vi "EXPRESS Launcher.vi"() -> ()   [LabVIEW 2010]
uses:
  Ctrls/Precess Meter.ctl
  Ctrls/PlotGraph.ctl
  Ctrls/ChannelData.ctl
  Ctrls/ChannelType.ctl
  Ctrls/ChannelAccessType.ctl
  Ctrls/ServerData.ctl
  Ctrls/DeviceInfomation.ctl
  Ctrls/DeviceModel.ctl
  Drivers/ModbusServer/MonitorServer.lvlib
panel:
  in  "剖面管理":bool
  in  "参数配置":bool
  in  "试验箱选择":i32(listbox)
  out "Waveform Graph":T1
  in  "ProcessMeter 4":T2 {"设定值" format="%07.2f"; "当前值" format="%07.2f"}
  in  "ProcessMeter 3":T2 {"设定值" format="%07.2f"; "当前值" format="%07.2f"}
  in  "ProcessMeter 2":T2 {"设定值" format="%07.2f"; "当前值" format="%07.2f"}
  in  "ProcessMeter 1":T2 {"设定值" format="%07.2f"; "当前值" format="%07.2f"}
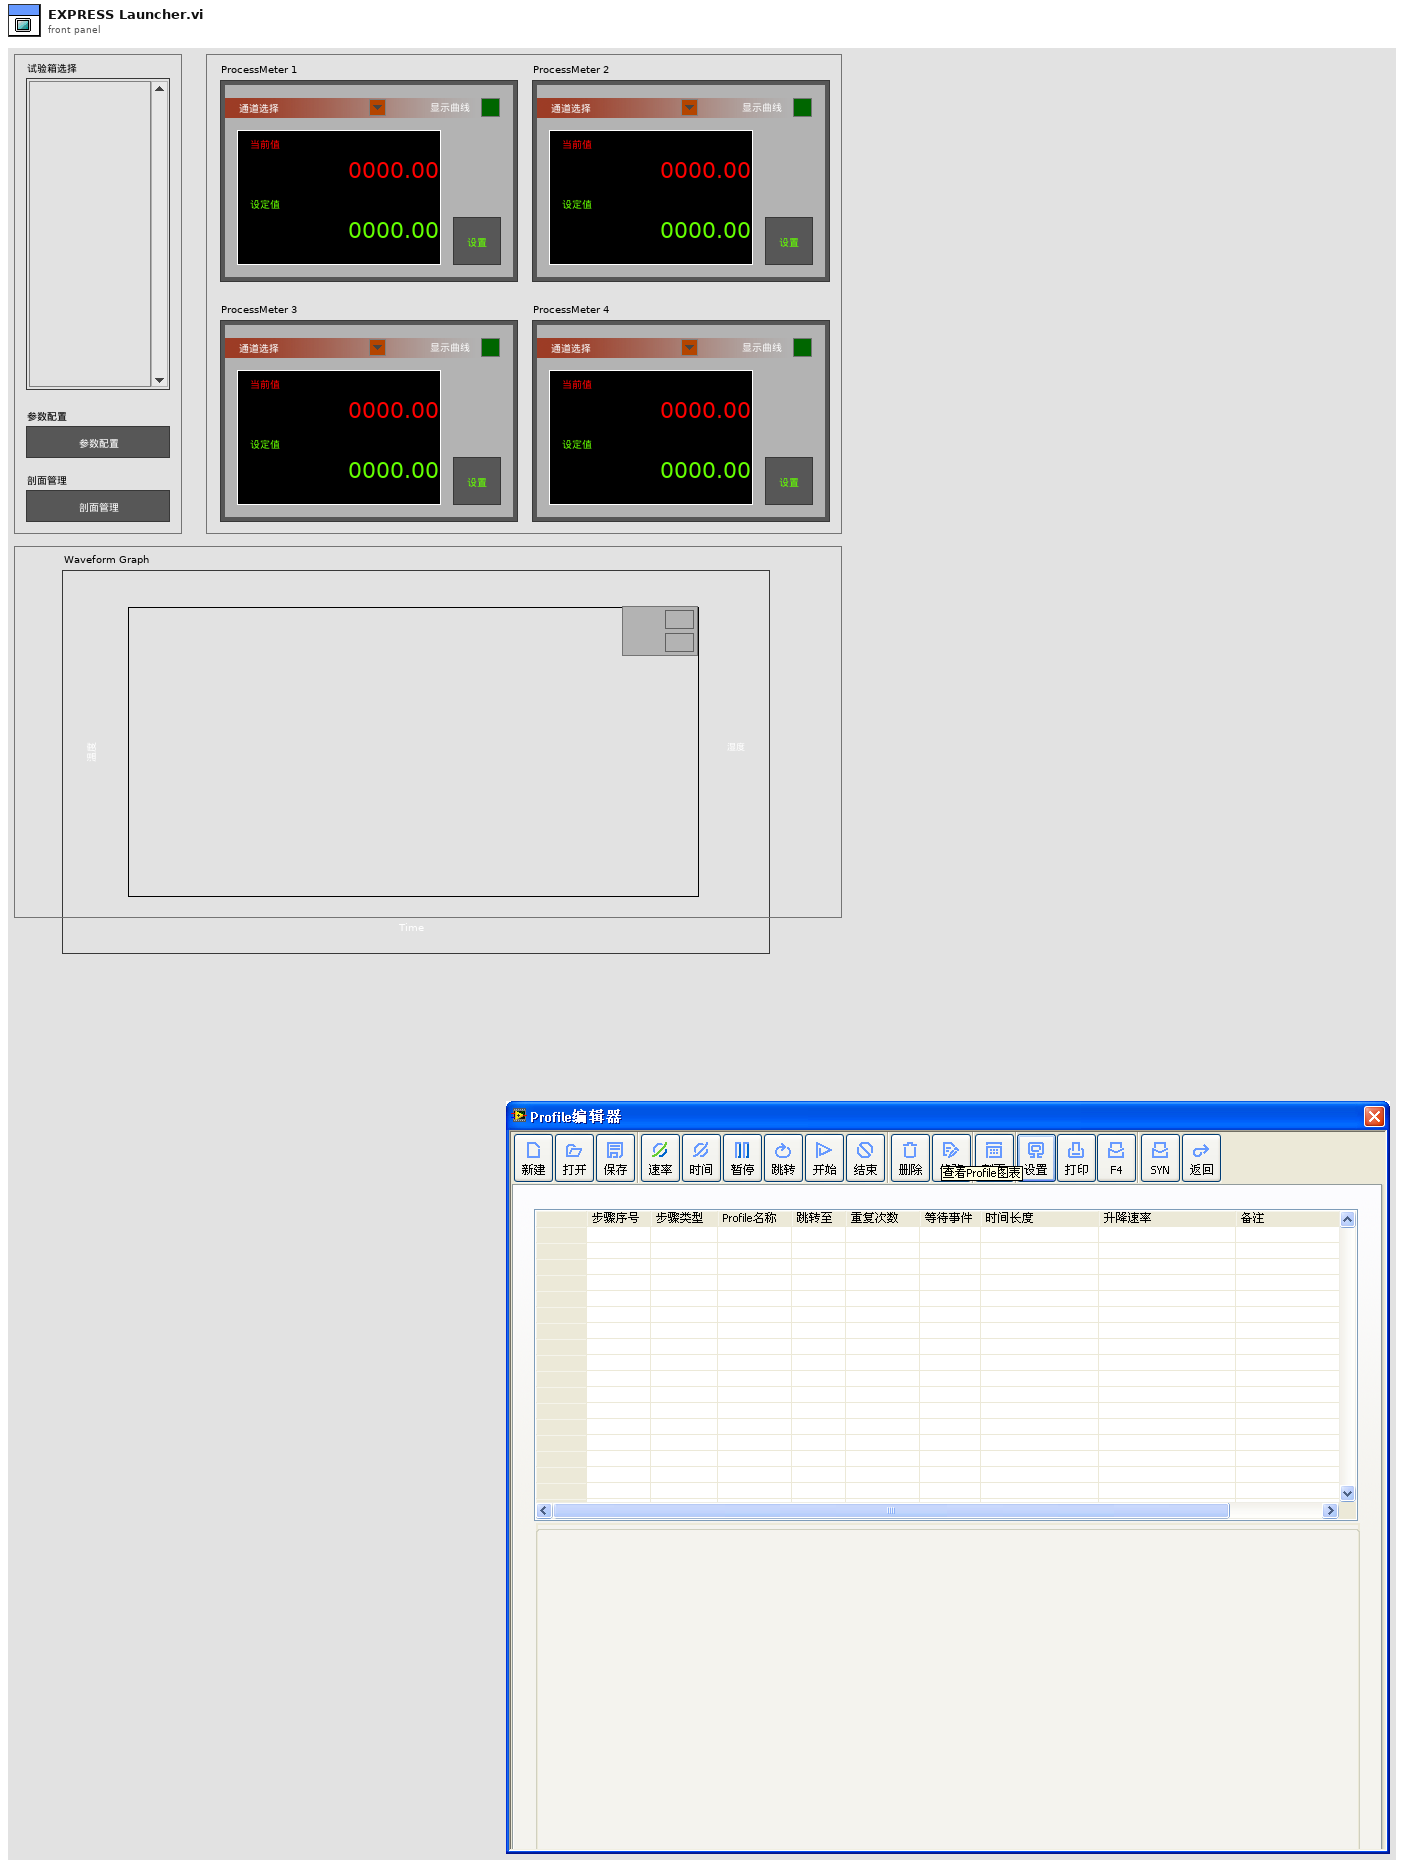
[diagram p1: front panel]
types:
  T1 = typedef "PlotGraph.ctl" = dbl[]
  T2 = typedef "Precess Meter.ctl" = cluster{"当前值":dbl, "设定值":dbl, "通道选择":string, "设置设定值":bool, "显示曲线":bool}
  T3 = enum8{"Enabled", "Disabled", "Disabled and Grayed Out"}
  T4 = enum32{"invalid app kind", "Development System", "Run Time System", "Student Edition", "Embedded LabVIEW", "Evaluation", "Custom"}
  T5 = typedef "ServerData.ctl" = T6[]
  T6 = typedef "DeviceInfomation.ctl" = cluster{"Model":T7, "ChamberName":string, "ChannelNumber":i32, "ChannelsData":T8[], "Connected":bool}
  T7 = typedef "DeviceModel.ctl" = enum16{"WatlowF4", "CenterOne", "DCP551", "DPR250"}
  T8 = typedef "ChannelData.ctl" = cluster{"ChannelName":string, "ChannelType":T9, "AccessType":T10, "ProcessValue":dbl, "SetValue":dbl, "NewSettValue":dbl, "SetNewTarget":bool}
  T9 = typedef "ChannelType.ctl" = enum16{"Temperature", "Humidity"}
  T10 = typedef "ChannelAccessType.ctl" = enum16{"ReadOnly", "SetTarget"}
  T11 = enum32{"Invalid", "Standard", "Closed", "Hidden", "Minimized", "Maximized"}
  T12 = cluster{"Core":cluster{"Current VI Reference":refnum<vi>, "Close Panel on Exit?":bool}, "SelectedDeviceChannelsData":T8[], "试验箱选择ref":refnum<vi>, "通道选择ref":refnum<vi>[], "ProcessMeterRef":refnum<vi>[]}
  T13 = cluster{"Current VI Reference":refnum<vi>, "Close Panel on Exit?":bool}
  T14 = typedef "Path InitDynamicVIsPaths__FS.ctl" = cluster{"F4 Operation":path, "F4 Alarms":path, "F4 Inputs":path, "F4 Outputs":path, "F4 PID Sets":path, "F4 Cascade":path, "F4 Current Step":path, "Profile SubPanel":path, "Profile Editor":path, "MainVI":path, "Profile Control":path, "Synergy Control":path, "Driver Server":path}
  T15 = typedef "Path InitPaths__FS.ctl" = cluster{"Ctrller CFG":path, "INI":path, "Profile":path, "EventLog":path, "Data":path}
  T16 = typedef "Controller Configuration__CHC.ctl" = cluster{"Ctrller Type":T17, "Ctrller Name":string, "Ctrller Addr":string, "Server IP":string, "Conn Result":string, "Port":string, "Baud":dbl}
  T17 = typedef "Controller Configuration__Ctrller Type.ctl" = enum16{"F4S/D", "Synergy"}
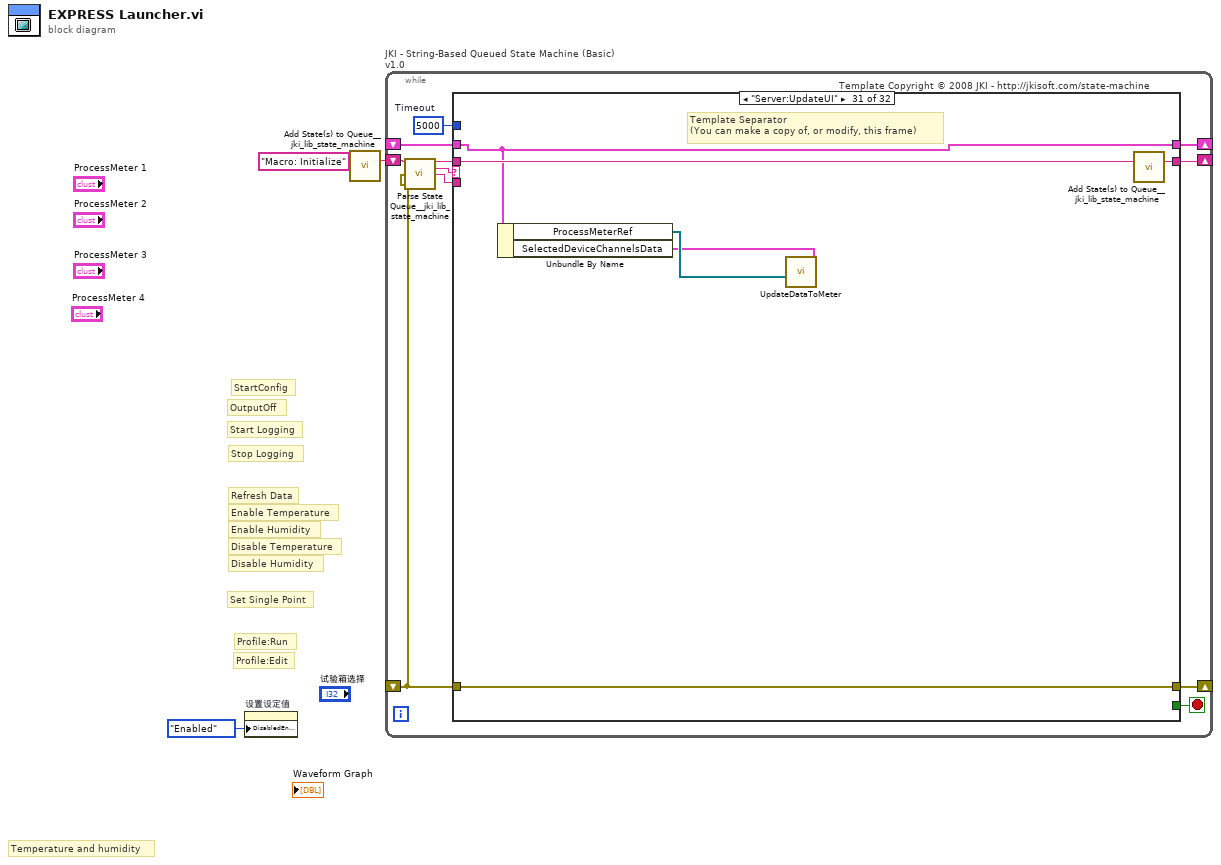
[diagram p0: block diagram]
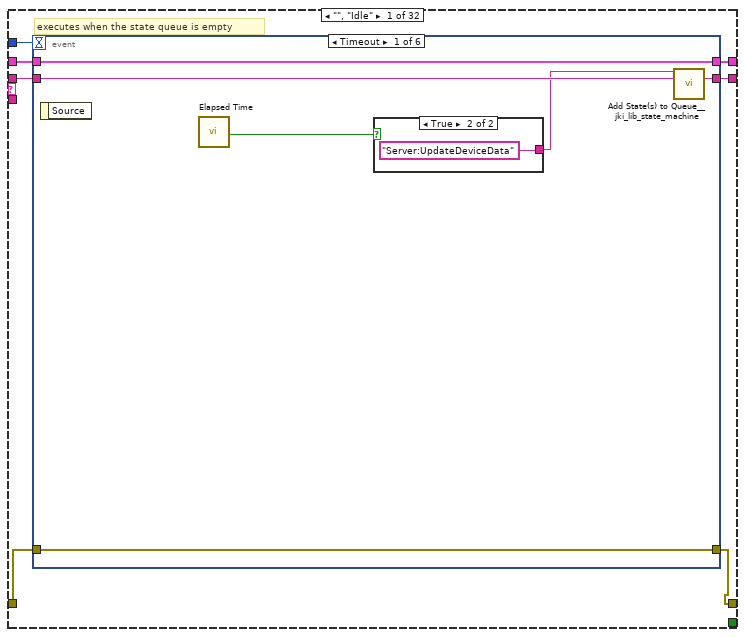
[diagram p2: hidden frame]
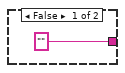
[diagram p3: hidden frame]
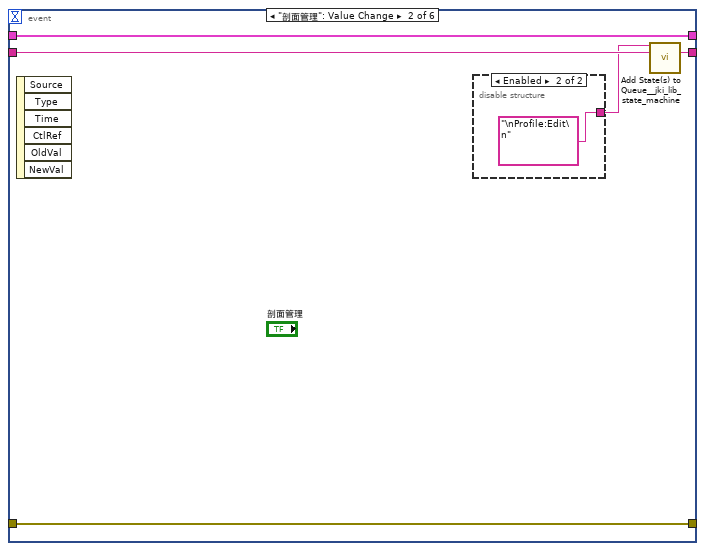
[diagram p4: hidden frame]
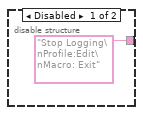
[diagram p5: hidden frame]
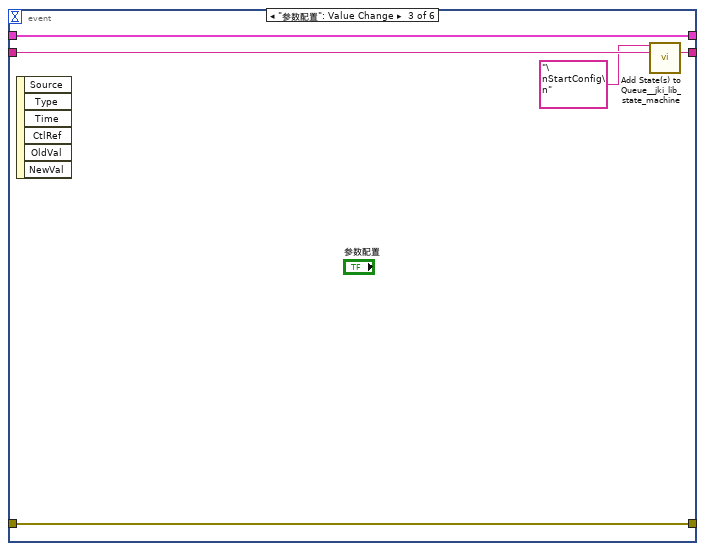
[diagram p6: hidden frame]
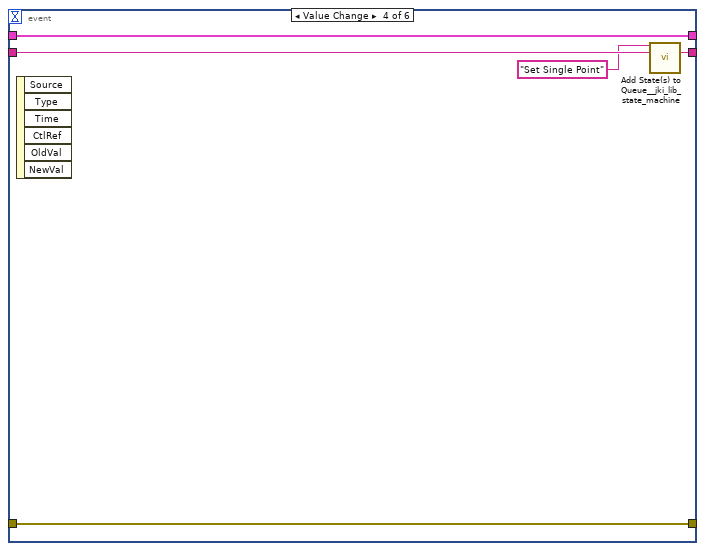
[diagram p7: hidden frame]
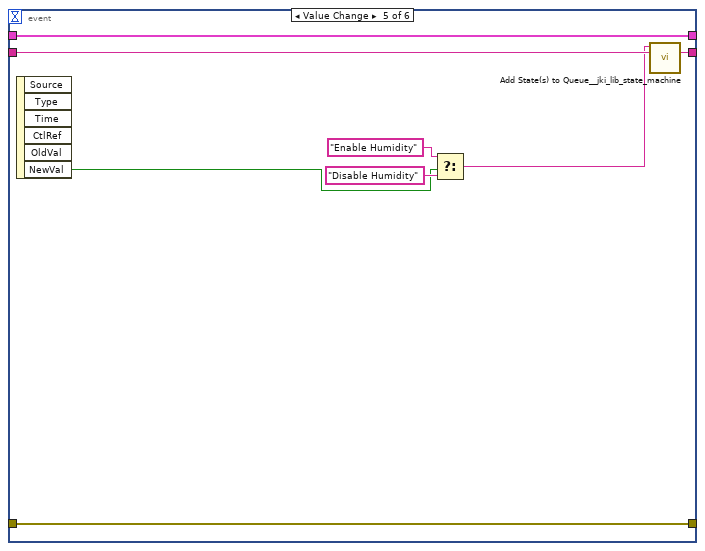
[diagram p8: hidden frame]
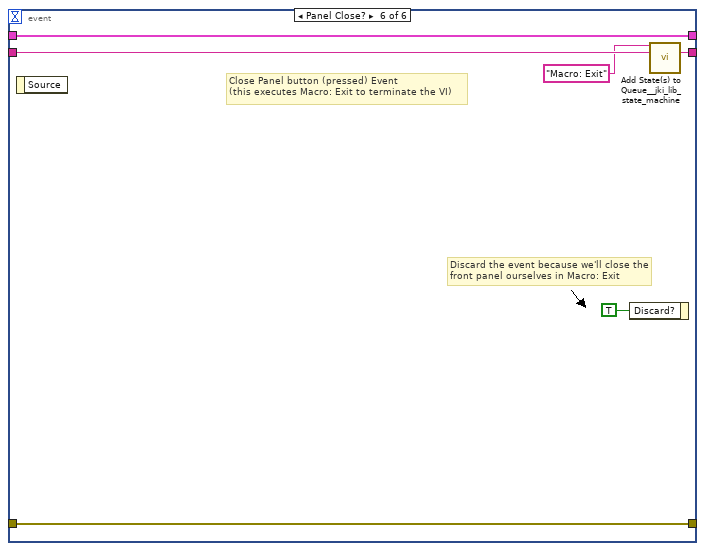
[diagram p9: hidden frame]
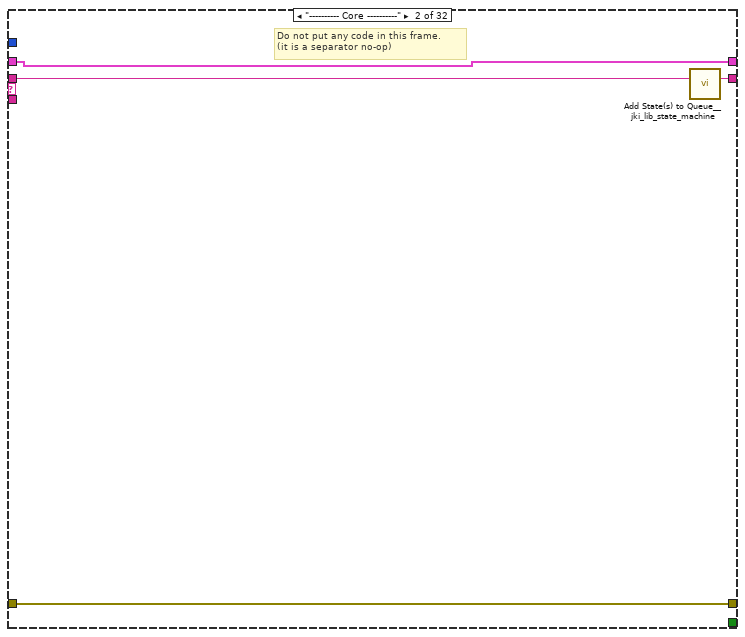
[diagram p10: hidden frame]
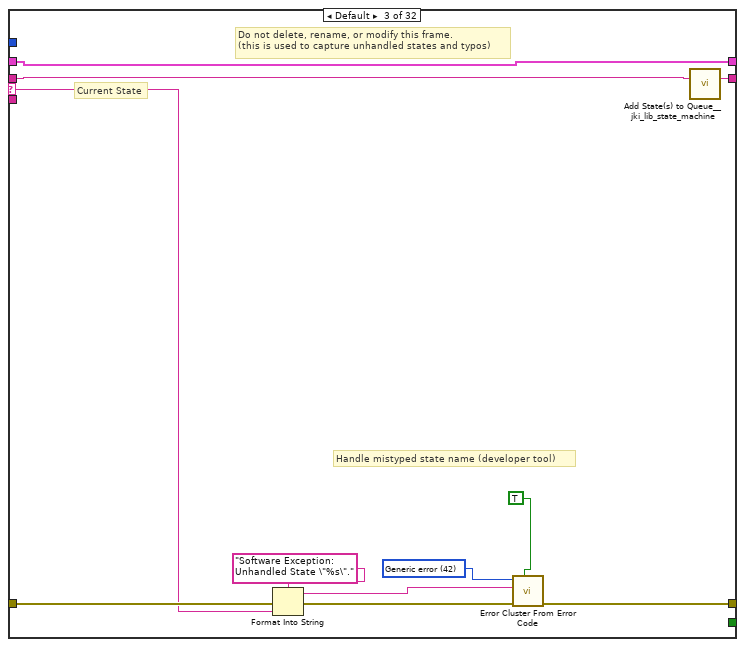
[diagram p11: hidden frame]
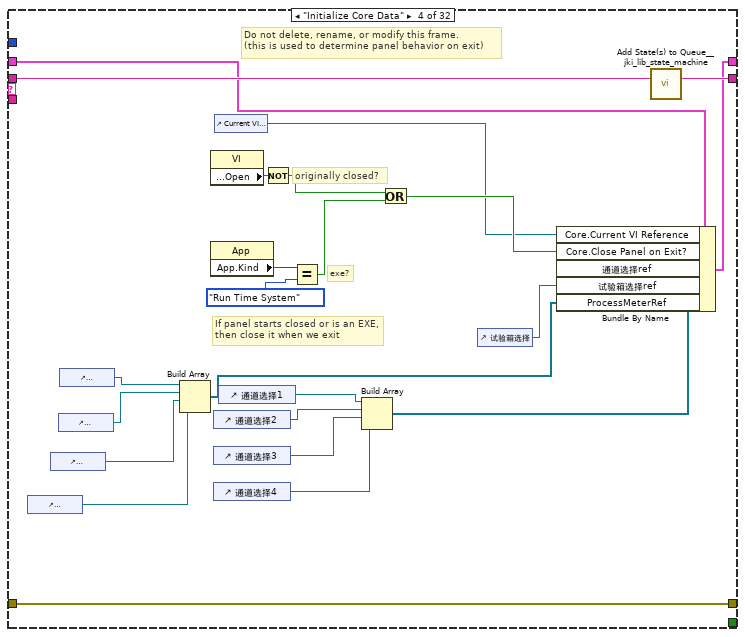
[diagram p12: hidden frame]
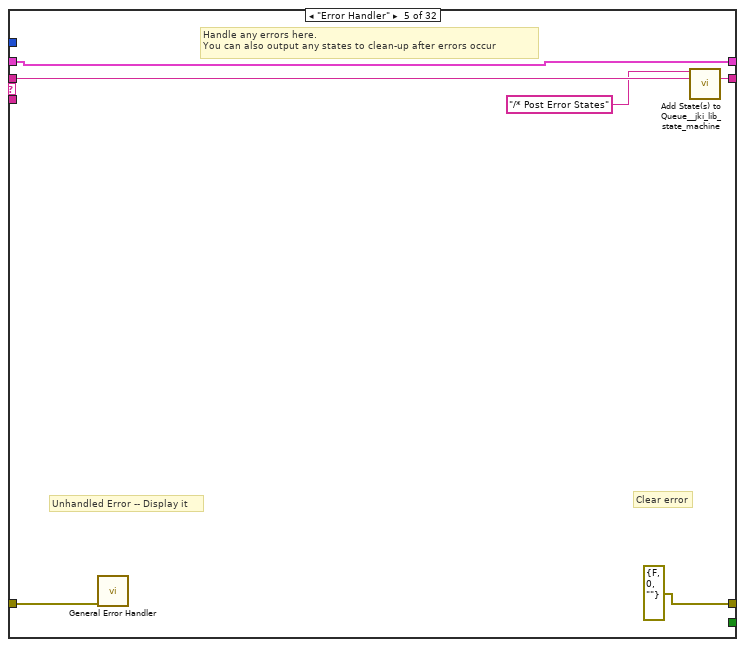
[diagram p13: hidden frame]
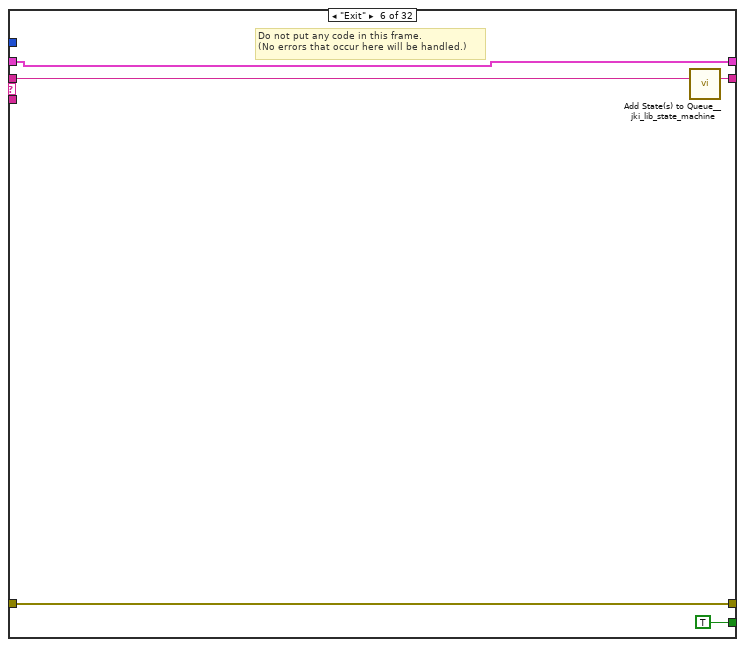
[diagram p14: hidden frame]
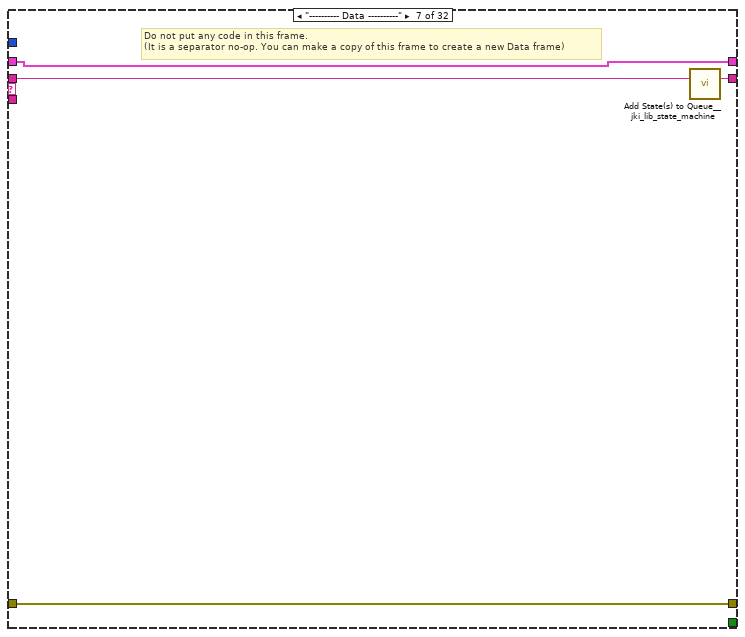
[diagram p15: hidden frame]
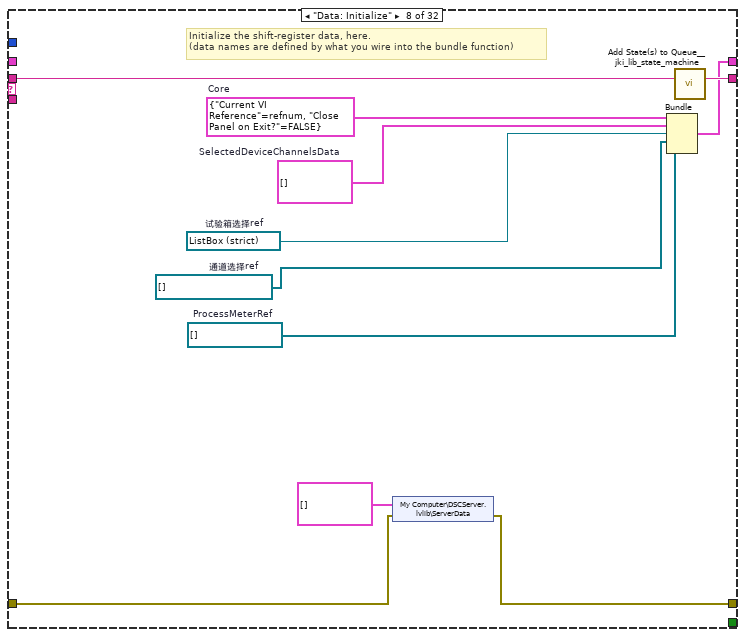
[diagram p16: hidden frame]
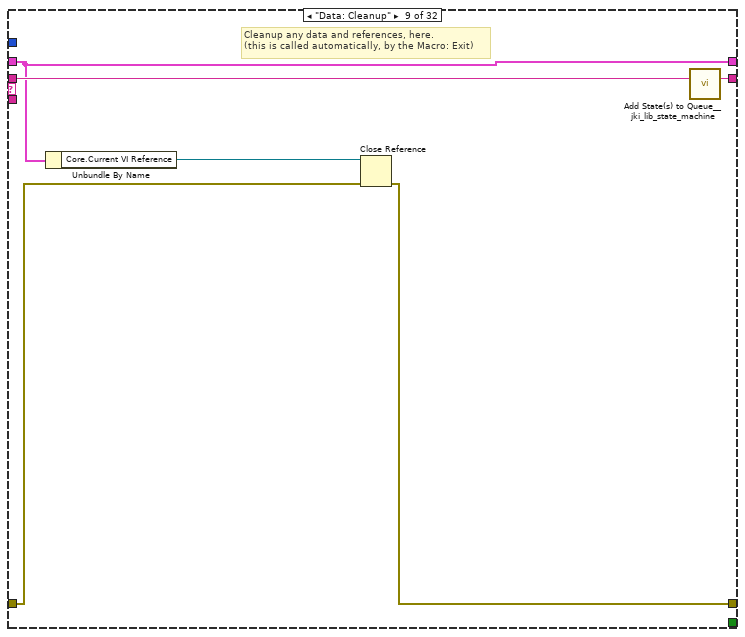
[diagram p17: hidden frame]
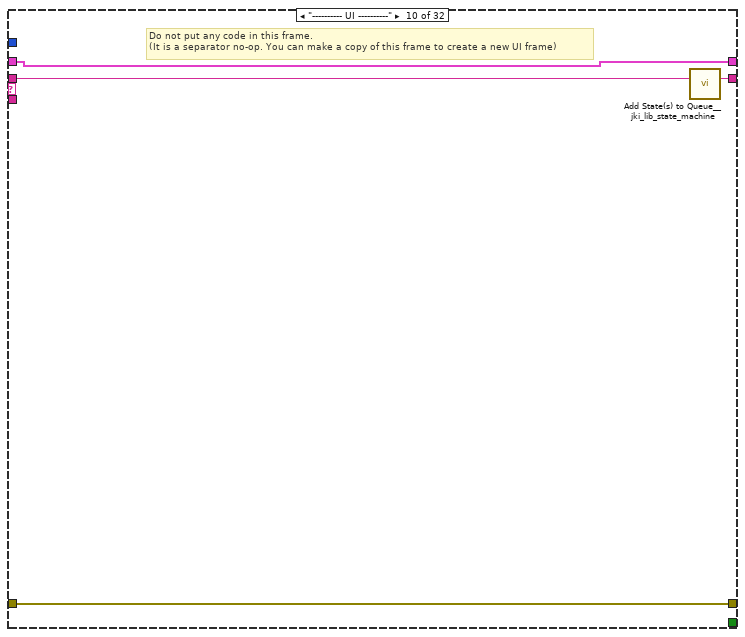
[diagram p18: hidden frame]
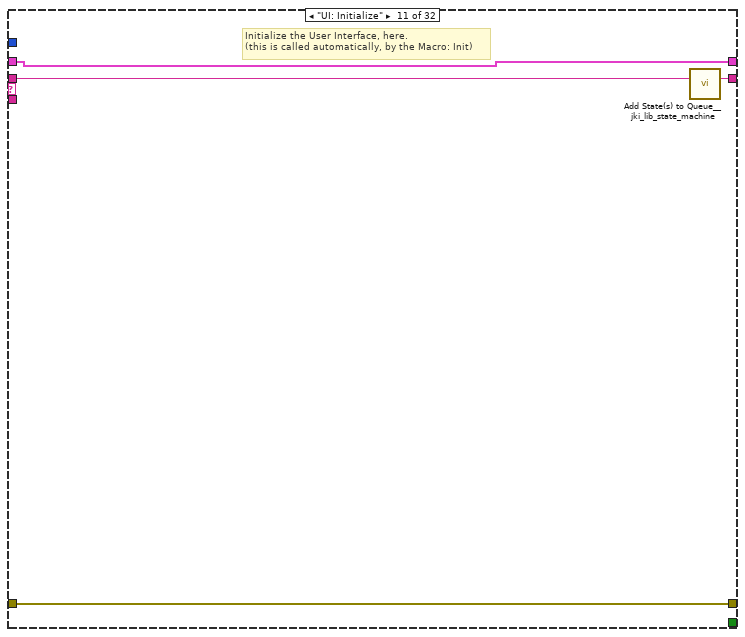
[diagram p19: hidden frame]
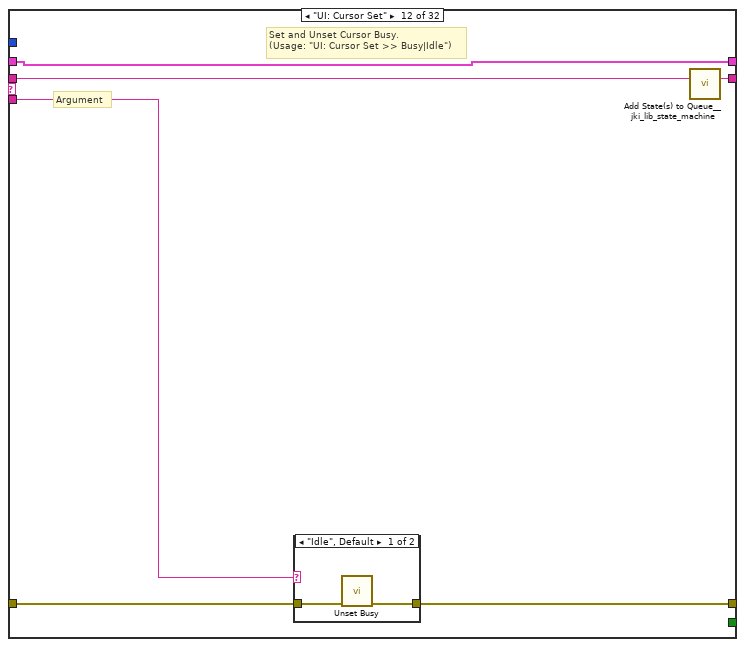
[diagram p20: hidden frame]
diagram:
  # "StartConfig"
  # "OutputOff"
  # "Profile:Edit"
  # "Profile:Run"
  # "Set Single Point"
  # "Stop Logging"
  # "Start Logging"
  # "Disable Humidity"
  # "Disable Temperature"
  # "Enable Temperature"
  # "Refresh Data"
  # "Enable Humidity"
  # "Temperature and humidity"
  n1 = property on="设置设定值" class="Bool"("DisabledEnum"=T3."Enabled" ("Disabled")) -> ()  [unwired: 2 in, 2 out]
  n2 = call "Add State(s) to Queue__jki_lib_state_machine.vi"("State(s) in (\"\")"="Macro: Initialize") -> ("States Out"=w3:string)  [unwired: 14 in]
  n3 = while "JKI - String-Based Queued State Machine (Basic) v1.0" {
    shift-right: [w7] -> _
    shift-left: _ -> [w6]
    shift-right: [w10] -> _
    shift-left: _ -> [w4]
    shift-right: [w9] -> _
    shift-left: w3 -> [w11]
    stop <- w8 stop-if-true
    w5 = 5000  # Timeout
    # "Template Copyright © 2008 JKI - http://jkisoft.com/state-machine"
    n4 = call "Parse State Queue__jki_lib_state_machine.vi"("State Queue"=w11, "Error In (no error)"=w4) -> ("Remaining States"=w13:string, "Current State"=w14:string, "Arguments"=w12:string)  [unwired: 11 in]
    n5 = case shown="\"Server:UpdateUI\"" w14 {
      selector: w14 -> [_ _ w65 _ _ _ _ _ _ _ _ _ _ _ _ _ _ _ _ _ _ _ _ _ _ _ _ _ _ _ _ _]
      tunnel: w13 -> [w21 w64 w69 w98 w104 w109 w113 w124 w130 w134 w138 w144 w155 w181 w186 w196 w200 w209 w214 w219 w227 w231 w236 w252 w257 w261 w265 w269 w273 w277 w283 w294]
      tunnel: w12 -> [_ _ _ _ _ _ _ _ _ _ _ w139 w149 _ _ _ _ _ _ _ _ _ _ _ _ _ _ _ _ _ _ _]
      tunnel: w6 -> [w19 w61 w67 w89 w101 w107 w110 _ w125 w131 w136 w142 w151 w178 w183 w193 w197 w207 w212 w217 w224 w228 w234 w250 w255 w259 w263 w267 w271 w274 w280 w291]
      tunnel: [w18 w62 w71 w95 errorcluster {"status"=FALSE, "code"=0, "source"=""} ("error out") w106 w111 w118 w126 w132 w135 w140 w152 w179 w184 w194 w198 w201 w210 w215 w225 w229 w232 w237 w253 w258 w262 w266 w270 w275 w281 w284] -> w10
      tunnel: w4 -> [w17 w62 w70 w95 w100 w106 w111 w119 w127 w132 w135 w141 w153 w179 w184 w194 w198 w202 w211 w216 w225 w229 w233 w241 w254 w258 w262 w266 w270 w275 w281 w285]
      tunnel: [w20 w63 w68 w97 w103 w108 w112 w123 w129 w133 w137 w143 w154 w180 w185 w195 w199 w208 w213 w218 w226 w230 w235 w251 w256 w260 w264 w268 w272 w276 w282 w293] -> w9
      tunnel: [_ _ _ _ _ TRUE _ _ _ _ _ _ _ _ _ _ _ _ _ _ _ _ _ _ _ _ _ _ _ _ _ _] -> w8
      tunnel: [w16 w61 w67 w96 w101 w107 w110 w122 w125 w131 w136 w142 w151 w178 w183 w193 w197 w207 w212 w217 w224 w228 w234 w250 w255 w259 w263 w267 w271 w274 w280 w287] -> w7
      tunnel: w5 -> [w15 _ _ _ _ _ _ _ _ _ _ _ _ _ _ _ _ _ _ _ _ _ _ _ _ _ _ _ _ _ _ _]
      frame "", "Idle" {
        # "executes when the state queue is empty"
        n6 = event shown="[0] Timeout" {
          selector: _ -> [_ _ _ _ _ _]
          dyn-events: _ -> [_ _ _ _ _ _]
          timeout: w15 -> [_ _ _ _ _ _]
          tunnel: w21 -> [w27 w34 w41 w46 w54 w60]
          tunnel: [w26 w33 w40 w45 w53 w59] -> w20
          tunnel: w19 -> [w24 w31 w38 w43 w51 w57]
          tunnel: [w25 w32 w39 w44 w52 w58] -> w18
          tunnel: w17 -> [w25 w32 w39 w44 w52 w58]
          tunnel: [w24 w31 w38 w43 w51 w57] -> w16
          event Timeout {
            n7 = event-data() -> ()  [unwired: 1 in, 1 out]
            n8 = call "Elapsed Time"() -> ("Time has Elapsed"=w23:bool)  [unwired: 12 in, 7 out]
            n9 = case shown="True" w23 {
              tunnel: ["" ("State(s) in Front (\"\")") "Server:UpdateDeviceData" ("State(s) in Front (\"\")")] -> w22
              frame False {
              }
              frame True {
              }
            }
            n10 = call "Add State(s) to Queue__jki_lib_state_machine.vi"("State(s) in Front (\"\")"=w22, "State(s) in (\"\")"=w27) -> ("States Out"=w26:string)  [unwired: 13 in]
          }
          event "剖面管理": Value Change {
            n11 = event-data() -> ()  [unwired: 1 in, 6 out]
            n12 = disable-structure shown="Enabled" {
              disable-tunnel: ["Stop Logging\nProfile:Edit\nMacro: Exit" ("State(s) in Front (\"\")") "\nProfile:Edit\n" ("State(s) in Front (\"\")")] -> w30
              frame Disabled {
              }
              frame Enabled {
              }
            }
            n13 = call "Add State(s) to Queue__jki_lib_state_machine.vi"("State(s) in Front (\"\")"=w30, "State(s) in (\"\")"=w34) -> ("States Out"=w33:string)  [unwired: 13 in]
          }
          event "参数配置": Value Change {
            n14 = event-data() -> ()  [unwired: 1 in, 6 out]
            n15 = call "Add State(s) to Queue__jki_lib_state_machine.vi"("State(s) in Front (\"\")"="\nStartConfig\n" ("State(s) in Front (\"\")"), "State(s) in (\"\")"=w41) -> ("States Out"=w40:string)  [unwired: 13 in]
          }
          event Value Change {
            n16 = event-data() -> ()  [unwired: 1 in, 6 out]
            n17 = call "Add State(s) to Queue__jki_lib_state_machine.vi"("State(s) in Front (\"\")"="Set Single Point" ("State(s) in Front (\"\")"), "State(s) in (\"\")"=w46) -> ("States Out"=w45:string)  [unwired: 13 in]
          }
          event Value Change {
            n18 = event-data() -> ("NewVal"=w47:bool)  [unwired: 1 in, 5 out]
            n19 = Select(t="Enable Humidity" ("State(s) in Front (\"\")"), s=w47, f="Disable Humidity") -> (s? t:f=w48:string)
            n20 = call "Add State(s) to Queue__jki_lib_state_machine.vi"("State(s) in Front (\"\")"=w48, "State(s) in (\"\")"=w54) -> ("States Out"=w53:string)  [unwired: 13 in]
          }
          event Panel Close? {
            # "Discard the event because we'll close the front panel ourselves in Macro: Exit"
            # "Close Panel button (pressed) Event\n(this executes Macro: Exit to terminate the VI)"
            n21 = event-data() -> ()  [unwired: 1 in, 1 out]
            n22 = event-data("Discard?"=TRUE) -> ()  [unwired: 1 in, 1 out]
            n23 = call "Add State(s) to Queue__jki_lib_state_machine.vi"("State(s) in Front (\"\")"="Macro: Exit", "State(s) in (\"\")"=w60) -> ("States Out"=w59:string)  [unwired: 13 in]
          }
        }
      }
      frame "---------- Core ----------" {
        # "Do not put any code in this frame.\n(it is a separator no-op)"
        n24 = call "Add State(s) to Queue__jki_lib_state_machine.vi"("State(s) in (\"\")"=w64) -> ("States Out"=w63:string)  [unwired: 14 in]
      }
      frame Default {
        w74 = 42 items=["No error", "Argument error", "Memory is full", "Out of zone", "End of file", "File already open", "Generic file I/O error", "File not found", "File permission error", "Disk is full", "Duplicate path", "Too many files open", "System feature not enabled", "Resource file not found", "Cannot add resource", "Resource not found", "Image not found", "Image memory error", "Pen does not exist", "Config type invalid", "Config token not found", "Config parse error", "Config memory error", "Bad external code format", "Bad external code offset", "External code not present", "Null window", "Destroy window error", "Null menu", "Print aborted", "Bad print record", "Print driver error", "Windows error during printing", "Memory error during printing", "Print dialog error", "Generic print error", "Invalid device refnum", "Device not found", "Device parameter error", "Device unit error", "Cannot open device", "Device call aborted", "Generic error", "Cancelled by user", "Object ID too low", "Object ID too high", "Object not in heap", "Unknown heap", "Unknown object (invalid DefProc)", "Unknown object (DefProc not in table)", "Message out of range", "Invalid (null) method", "Unknown message", "Manager call not supported", "Bad address", "Network operation in progress", "Network operation timed out", "Connection is busy", "Network attribute not supported", "Network error", "Address in use", "System out of memory", "Connection aborted", "Connection refused", "Not connected", "Already connected", "Connection closed", "Initialization error (interapplication manager)", "Bad occurrence", "Wait on unbound occurrence handler", "Occurrence queue overflow", "Datalog type conflict", "Unused", "Unrecognized type (interapplication manager)", "Memory corrupt", "Failed to make temporary DLL", "Old CIN version", "Drag socket not found", "Failed to load drop-object", "Failed to register OLE object", "Failed to release OLE object", "Format specifier type mismatch", "Unknown format specifier", "Too few format specifiers", "Too many format specifiers", "Scan failed", "Newer CIN version", "Error converting to variant", "Runtime menu error", "Password tampered", "Variant attribute not found", "Incompatible variant data type", "Event data is not available", "Event Store is not present", "Occurrence is not found", "Event Queue is not created", "Event info is not available", "Refnum passed is NULL", "Error retrieving Class GUID", "Error retrieving CoClass GUID", "Error retrieving TypeLib GUID.", "Bad built application magic bytes.", "Specific driver is different from the specific driver associated with the Logical Name.", "There is no session opened to the class driver.", "Max Error", "MAX - Error with config objects", "MAX - Error loading configuration", "MAX - Group not supported"]
        # "Current State"
        # "Do not delete, rename, or modify this frame.\n(this is used to capture unhandled states and typos)"
        # "Handle mistyped state name (developer tool)"
        n25 = Format Into String(format string="Software Exception: Unhandled State \"%s\"." ("message"), error in=w70, w65) -> (resulting string=w73:string, error out=w72:errorcluster)  [unwired: 1 in]
        n26 = call <vilib>:"Error Cluster From Error Code.vi"("show call chain? (False)"=TRUE, "error in (no error)"=w72, "error message (\"\")"=w73, "error code (0)"=w74) -> ("error out"=w71:errorcluster)  [unwired: 5 in]
        n27 = call "Add State(s) to Queue__jki_lib_state_machine.vi"("State(s) in (\"\")"=w69) -> ("States Out"=w68:string)  [unwired: 14 in]
      }
      frame "Initialize Core Data" {
        # "Do not delete, rename, or modify this frame.\n(this is used to determine panel behavior on exit)"
        # "originally closed?"
        # "exe?"
        # "If panel starts closed or is an EXE, then close it when we exit"
        n28 = control-ref of="ProcessMeter 4"() -> (w77:refnum<vi>)
        n29 = control-ref of="ProcessMeter 3"() -> (w78:refnum<vi>)
        n30 = control-ref of="ProcessMeter 2"() -> (w79:refnum<vi>)
        n31 = control-ref of="ProcessMeter 1"() -> (w80:refnum<vi>)
        n32 = Build Array(w80, w79, w78, w77) -> (w76:refnum<vi>[])
        n33 = property class="VI"() -> ("Front Panel.Open"=w94:bool)  [unwired: 2 in, 2 out]
        n34 = property class="App"() -> ("App.Kind"=w93:T4)  [unwired: 2 in, 2 out]
        n35 = control-ref of="通道选择2"() -> (w85:refnum<vi>)
        n36 = control-ref of="通道选择3"() -> (w84:refnum<vi>)
        n37 = control-ref of="通道选择4"() -> (w83:refnum<vi>)
        n38 = control-ref of="Current VI Reference"() -> (w87:refnum<vi>)
        n39 = control-ref of="通道选择1"() -> (w86:refnum<vi>)
        n40 = Not(x=w94) -> (.not. x?=w91:bool)
        n41 = Equal?(x=w93, y=T4."Run Time System" ("Application:Kind")) -> (x = y?=w90:bool)
        n42 = Build Array(w86, w85, w84, w83) -> (w82:refnum<vi>[])
        n43 = Or(x=w91, y=w90) -> (x .or. y?=w88:bool)
        n44 = control-ref of="试验箱选择"() -> (w81:refnum<vi>)
        n45 = Bundle By Name(cluster=w89, "Core.Current VI Reference"=w87, "Core.Close Panel on Exit?"=w88, "通道选择ref"=w82, "试验箱选择ref"=w81, "ProcessMeterRef"=w76) -> (w96:T12)
        n46 = call "Add State(s) to Queue__jki_lib_state_machine.vi"("State(s) in (\"\")"=w98) -> ("States Out"=w97:string)  [unwired: 14 in]
      }
      frame "Error Handler" {
        # "Unhandled Error -- Display it"
        # "Handle any errors here.\nYou can also output any states to clean-up after errors occur"
        # "Clear error"
        n47 = call <vilib>:"General Error Handler.vi"("error in (no error)"=w100) -> ()  [unwired: 10 in, 5 out]
        n48 = call "Add State(s) to Queue__jki_lib_state_machine.vi"("State(s) in Front (\"\")"="/* Post Error States", "State(s) in (\"\")"=w104) -> ("States Out"=w103:string)  [unwired: 13 in]
      }
      frame "Exit" {
        # "Do not put any code in this frame.\n(No errors that occur here will be handled.)"
        n49 = call "Add State(s) to Queue__jki_lib_state_machine.vi"("State(s) in (\"\")"=w109) -> ("States Out"=w108:string)  [unwired: 14 in]
      }
      frame "---------- Data ----------" {
        # "Do not put any code in this frame.\n(It is a separator no-op. You can make a copy of this frame to create a new Data frame)"
        n50 = call "Add State(s) to Queue__jki_lib_state_machine.vi"("State(s) in (\"\")"=w113) -> ("States Out"=w112:string)  [unwired: 14 in]
      }
      frame "Data: Initialize" {
        w114 = refnum<vi>[] []  # ProcessMeterRef
        w115 = refnum<vi> refnum  # 试验箱选择ref
        w116 = refnum<vi>[] []  # 通道选择ref
        w117 = T8[] []  # SelectedDeviceChannelsData
        w121 = T13 {"Current VI Reference"=refnum, "Close Panel on Exit?"=FALSE}  # Core
        # "Initialize the shift-register data, here.\n(data names are defined by what you wire into the bundle function)"
        n51 = shared-variable "My Computer\\DSCServer.lvlib\\ServerData"(T5 [] ("ServerData"), error in=w119) -> (error out=w118:errorcluster)
        n52 = Bundle("Core"=w121, "SelectedDeviceChannelsData"=w117, "试验箱选择ref"=w115, "通道选择ref"=w116, "ProcessMeterRef"=w114) -> (w122:T12)  [unwired: 1 in]
        n53 = call "Add State(s) to Queue__jki_lib_state_machine.vi"("State(s) in (\"\")"=w124) -> ("States Out"=w123:string)  [unwired: 14 in]
      }
      frame "Data: Cleanup" {
        # "Cleanup any data and references, here.\n(this is called automatically, by the Macro: Exit)"
        n54 = Unbundle By Name(w125) -> ("Core.Current VI Reference"=w128:refnum<vi>)
        n55 = Close Reference(reference=w128, error in (no error)=w127) -> (error out=w126:errorcluster)
        n56 = call "Add State(s) to Queue__jki_lib_state_machine.vi"("State(s) in (\"\")"=w130) -> ("States Out"=w129:string)  [unwired: 14 in]
      }
      frame "---------- UI ----------" {
        # "Do not put any code in this frame.\n(It is a separator no-op. You can make a copy of this frame to create a new UI frame)"
        n57 = call "Add State(s) to Queue__jki_lib_state_machine.vi"("State(s) in (\"\")"=w134) -> ("States Out"=w133:string)  [unwired: 14 in]
      }
      frame "UI: Initialize" {
        # "Initialize the User Interface, here.\n(this is called automatically, by the Macro: Init)"
        n58 = call "Add State(s) to Queue__jki_lib_state_machine.vi"("State(s) in (\"\")"=w138) -> ("States Out"=w137:string)  [unwired: 14 in]
      }
      frame "UI: Cursor Set" {
        # "Argument"
        # "Set and Unset Cursor Busy.\n(Usage: \"UI: Cursor Set >> Busy|Idle\")"
        n59 = case shown="\"Idle\", Default" w139 {
          tunnel: w141 -> [w146 w148]
          tunnel: [w145 w147] -> w140
          frame "Idle", Default {
            n60 = call <vilib>:"Unset Busy.vi"("error in (no error)"=w146) -> ("error out"=w145:errorcluster)  [unwired: 10 in]
          }
          frame "Busy" {
            n61 = call <vilib>:"Set Busy.vi"("error in (no error)"=w148) -> ("error out"=w147:errorcluster)  [unwired: 9 in, 1 out]
          }
        }
        n62 = call "Add State(s) to Queue__jki_lib_state_machine.vi"("State(s) in (\"\")"=w144) -> ("States Out"=w143:string)  [unwired: 14 in]
      }
      frame "UI: Front Panel State" {
        # "Argument"
        # "Set Front Panel Open or Closed\n(Usage: \"UI: Front Panel State >> Open|Close\")"
        n63 = Unbundle By Name(w151) -> ("Core.Current VI Reference"=w150:refnum<vi>)
        n64 = case shown="\"Open\", Default" w149 {
          tunnel: w153 -> [w159 w172]
          tunnel: [w161 w173] -> w152
          tunnel: w150 -> [w160 w170]
          frame "Open", Default {
            n65 = property class="VI"(reference=w160, error in=w159) -> (reference out=w157:refnum<vi>, error out=w158:errorcluster, "Front Panel.Open"=w156:bool)
            n66 = case shown="False" w156 {
              tunnel: [w164 w167] -> w161
              tunnel: w158 -> [w163 w167]
              tunnel: w157 -> [w162 _]
              frame False {
                n67 = invoke class="VI" method="FP.Open"(reference=w162, error in=w163, "Activate"=TRUE, "State"=T11."Standard") -> (error out=w164:errorcluster)  [unwired: 1 in, 4 out]
              }
              frame True {
              }
            }
          }
          frame "Close" {
            n68 = property class="VI"(reference=w170, error in=w172) -> (reference out=w169:refnum<vi>, error out=w171:errorcluster, "Front Panel.Open"=w168:bool)
            n69 = case shown="True" w168 {
              tunnel: [w174 w177] -> w173
              tunnel: w171 -> [w174 w176]
              tunnel: w169 -> [_ w175]
              frame False {
              }
              frame True {
                n70 = invoke class="VI" method="FP.Close"(reference=w175, error in=w176) -> (error out=w177:errorcluster)  [unwired: 1 in, 2 out]
              }
            }
          }
        }
        n71 = call "Add State(s) to Queue__jki_lib_state_machine.vi"("State(s) in (\"\")"=w155) -> ("States Out"=w154:string)  [unwired: 14 in]
      }
      frame "---------- Macro ----------" {
        # "Do not put any code in this frame.\n(It is a separator no-op. You can make a copy of this frame to create a new Macro frame)"
        n72 = call "Add State(s) to Queue__jki_lib_state_machine.vi"("State(s) in (\"\")"=w181) -> ("States Out"=w180:string)  [unwired: 14 in]
      }
      frame "Macro: Initialize" {
        w182 = "Data: Initialize\nInitialize Core Data\nUI: Initialize\nUI: Front Panel State >> Open\n\nServer:UpdateDeviceData"  # Data: Initialize Initialize Core Data UI: Initialize UI: Front Panel State >> Open  Server:UpdateDeviceData
        # "Initialization Macro\n(This is called once, when the VI starts)"
        n73 = call "Add State(s) to Queue__jki_lib_state_machine.vi"("State(s) in Front (\"\")"=w182, "State(s) in (\"\")"=w186) -> ("States Out"=w185:string)  [unwired: 13 in]
      }
      frame "Macro: Exit" {
        # "Exit Macro\n(This is called once, when the VI exits)"
        n74 = Unbundle By Name(w193) -> ("Core.Close Panel on Exit?"=w192:bool)
        n75 = Select(t="UI: Front Panel State >> Close", s=w192, f="") -> (s? t:f=w189:string)
        n76 = call "Add State(s) to Queue__jki_lib_state_machine.vi"("State(s) in (\"\")"=w189, "State(s) at Back (\"\")"="Stop Logging\nData: Cleanup\nExit") -> ("States Out"=w187:string)  [unwired: 13 in]
        n77 = call "Add State(s) to Queue__jki_lib_state_machine.vi"("State(s) in Front (\"\")"=w187, "State(s) in (\"\")"=w196) -> ("States Out"=w195:string)  [unwired: 13 in]
      }
      frame "---------- New Category ----------" {
        # "Template Separator\n(You can make a copy of, or modify, this frame)"
        n78 = call "Add State(s) to Queue__jki_lib_state_machine.vi"("State(s) in (\"\")"=w200) -> ("States Out"=w199:string)  [unwired: 14 in]
      }
      frame "StartConfig" {
        # "Template Separator\n(You can make a copy of, or modify, this frame)"
        n79 = call "File System Paths__FS.vi"("error in (no error)"=w202) -> ("error out"=w203:errorcluster, "DynamicVIs"=w206:T14)  [unwired: 8 in, 1 out]
        n80 = Unbundle By Name(w206) -> ("MainVI"=w205:path)
        n81 = call "Dynamic Call__Uti.vi"("error in (no error)"=w203, "open front panel? (T)"=TRUE, "vi path"=w205) -> ("error out"=w201:errorcluster)  [unwired: 8 in]
        n82 = call "Add State(s) to Queue__jki_lib_state_machine.vi"("State(s) in (\"\")"=w209) -> ("States Out"=w208:string)  [unwired: 14 in]
      }
      frame "OutputOff" {
        # "Template Separator\n(You can make a copy of, or modify, this frame)"
        n83 = call "OutPutOff.vi"("error in (no error)"=w211) -> ("error out"=w210:errorcluster)  [unwired: 10 in]
        n84 = call "Add State(s) to Queue__jki_lib_state_machine.vi"("State(s) in (\"\")"=w214) -> ("States Out"=w213:string)  [unwired: 14 in]
      }
      frame "Profile:Run" {
        # "Template Separator\n(You can make a copy of, or modify, this frame)"
        n85 = call "RunProfile.vi"("error in"=w216) -> ("error out"=w215:errorcluster)  [unwired: 10 in]
        n86 = call "Add State(s) to Queue__jki_lib_state_machine.vi"("State(s) in (\"\")"=w219) -> ("States Out"=w218:string)  [unwired: 14 in]
      }
      frame "Profile:Edit" {
        # "Template Separator\n(You can make a copy of, or modify, this frame)"
        n87 = call "File System Paths__FS.vi"() -> ("error out"=w220:errorcluster, "DynamicVIs"=w223:T14)  [unwired: 9 in, 1 out]
        n88 = Unbundle By Name(w223) -> ("Profile Editor"=w222:path)
        n89 = call "Dynamic Call__Uti.vi"("error in (no error)"=w220, "open front panel? (T)"=TRUE, "vi path"=w222) -> ()  [unwired: 8 in, 1 out]
        n90 = call "Add State(s) to Queue__jki_lib_state_machine.vi"("State(s) in (\"\")"=w227) -> ("States Out"=w226:string)  [unwired: 14 in]
      }
      frame "Set Single Point" {
        # "Template Separator\n(You can make a copy of, or modify, this frame)"
        n91 = disable-structure shown="Disabled" {
          frame Disabled {
            n92 = call "SetSinglePoint.vi"() -> ()  [unwired: 12 in]
          }
          frame Enabled {
          }
        }
        n93 = call "Add State(s) to Queue__jki_lib_state_machine.vi"("State(s) in (\"\")"=w231) -> ("States Out"=w230:string)  [unwired: 14 in]
      }
      frame "Stop Logging" {
        # "Template Separator\n(You can make a copy of, or modify, this frame)"
        n94 = call "StopServer.vi"("error in (no error)"=w233) -> ("error out"=w232:errorcluster)  [unwired: 10 in]
        n95 = call "Add State(s) to Queue__jki_lib_state_machine.vi"("State(s) in (\"\")"=w236) -> ("States Out"=w235:string)  [unwired: 14 in]
      }
      frame "Refresh Data" {
        w242 = 3600  # Datalength
        # "Your code here.\n(You can make a copy of, or modify, this frame)"
        n96 = call "File System Paths__FS.vi"() -> ("FilePaths"=w249:T15)  [unwired: 9 in, 2 out]
        n97 = Unbundle By Name(w249) -> ("Data"=w244:path, "Ctrller CFG"=w239:path)
        n98 = Build Path(base path=w244, name or relative path="default.tdms") -> (appended path=w243:path)
        n99 = call "Ctrller Cfg Read__FS.vi"("Path In"=w239) -> ("Ctrllers"=w248:T16[])  [unwired: 8 in, 2 out]
        n100 = Index Array(array=w248, index=0) -> (element=w246:T16)
        n101 = Unbundle By Name(w246) -> ("Ctrller Name"=w238:string)
        n102 = call "DataPlayback.vi"("error in (no error)"=w241, "Datalength"=w242, "Controller Name"=w238, "file path"=w243) -> ("error out"=w240:errorcluster)  [unwired: 6 in, 1 out]
        n103 = call <vilib>:"Clear Errors.vi"("error in (no error)"=w240) -> ("error out"=w237:errorcluster)  [unwired: 6 in]
        n104 = call "Add State(s) to Queue__jki_lib_state_machine.vi"("State(s) in (\"\")"=w252) -> ("States Out"=w251:string)  [unwired: 14 in]
      }
      frame "Start Logging" {
        # "Your code here.\n(You can make a copy of, or modify, this frame)"
        n105 = call "StartServer.vi"("error in (no error)"=w254) -> ("error out"=w253:errorcluster)  [unwired: 10 in]
        n106 = call "Add State(s) to Queue__jki_lib_state_machine.vi"("State(s) in (\"\")"=w257) -> ("States Out"=w256:string)  [unwired: 14 in]
      }
      frame "Enable Temperature" {
        # "Your code here.\n(You can make a copy of, or modify, this frame)"
        n107 = call "Add State(s) to Queue__jki_lib_state_machine.vi"("State(s) in (\"\")"=w261) -> ("States Out"=w260:string)  [unwired: 14 in]
      }
      frame "Enable Humidity" {
        # "Your code here.\n(You can make a copy of, or modify, this frame)"
        n108 = call "Add State(s) to Queue__jki_lib_state_machine.vi"("State(s) in (\"\")"=w265) -> ("States Out"=w264:string)  [unwired: 14 in]
      }
      frame "Disable Temperature" {
        # "Your code here.\n(You can make a copy of, or modify, this frame)"
        n109 = call "Add State(s) to Queue__jki_lib_state_machine.vi"("State(s) in (\"\")"=w269) -> ("States Out"=w268:string)  [unwired: 14 in]
      }
      frame "Disable Humidity" {
        # "Your code here.\n(You can make a copy of, or modify, this frame)"
        n110 = call "Add State(s) to Queue__jki_lib_state_machine.vi"("State(s) in (\"\")"=w273) -> ("States Out"=w272:string)  [unwired: 14 in]
      }
      frame "----------Server----------" {
        # "Template Separator\n(You can make a copy of, or modify, this frame)"
        n111 = call "Add State(s) to Queue__jki_lib_state_machine.vi"("State(s) in (\"\")"=w277) -> ("States Out"=w276:string)  [unwired: 14 in]
      }
      frame "Server:UpdateUI" {
        # "Template Separator\n(You can make a copy of, or modify, this frame)"
        n112 = Unbundle By Name(w280) -> ("ProcessMeterRef"=w279:refnum<vi>[], "SelectedDeviceChannelsData"=w278:T8[])
        n113 = call "UpdateDataToMeter.vi"("SelectedDeviceChannelsData"=w278, "ProcessMeterRef"=w279) -> ()  [unwired: 10 in]
        n114 = call "Add State(s) to Queue__jki_lib_state_machine.vi"("State(s) in (\"\")"=w283) -> ("States Out"=w282:string)  [unwired: 14 in]
      }
      frame "Server:UpdateDeviceData" {
        # "Template Separator\n(You can make a copy of, or modify, this frame)"
        n115 = Unbundle By Name(w291) -> ("Core.Current VI Reference"=w290:refnum<vi>, "试验箱选择ref"=w289:refnum<vi>, "通道选择ref"=w288:refnum<vi>[])
        n116 = shared-variable "My Computer\\DSCServer.lvlib\\ServerData"() -> (w292:T5)  [unwired: 1 in, 1 out]
        n117 = call "ParseServerData.vi"("通道选择ref"=w288, "error in (no error)"=w285, "试验箱选择"=w289, "This VI"=w290, "ServerData"=w292) -> ("error out"=w284:errorcluster, "SelectedDeviceChannelsData"=w286:T8[])  [unwired: 5 in]
        n118 = Bundle By Name(cluster=w291, "SelectedDeviceChannelsData"=w286) -> (w287:T12)
        n119 = call "Add State(s) to Queue__jki_lib_state_machine.vi"("State(s) in (\"\")"=w294) -> ("States Out"=w293:string)  [unwired: 14 in]
      }
    }
  }
